vi "initErrorList.vi"(8 "error in (no error)":errorcluster, 11 "Electrometer in":refnum<class "Electrometer.lvclass">) -> (0 "error out":errorcluster, 3 "Electrometer out":refnum<class "Electrometer.lvclass">)   [LabVIEW 2016, in "Electrometer.lvclass"]
uses:
  Electrometer.lvclass
  ElectrometerConfiguration/ElectrometerInternalConfiguration.lvclass
  ElectrometerError/ElectrometerError.lvclass
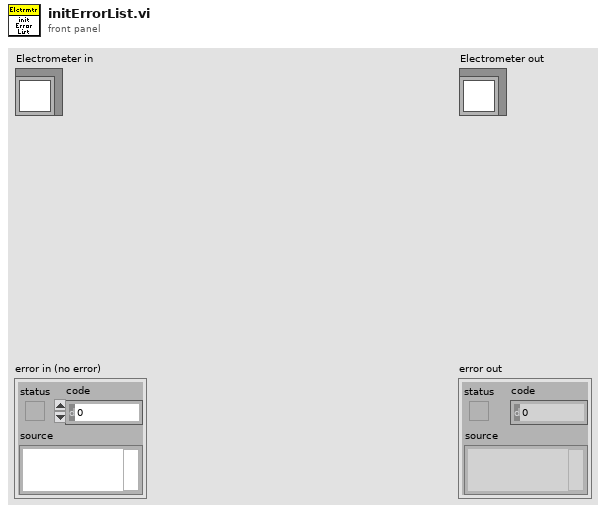
[diagram p1: front panel]
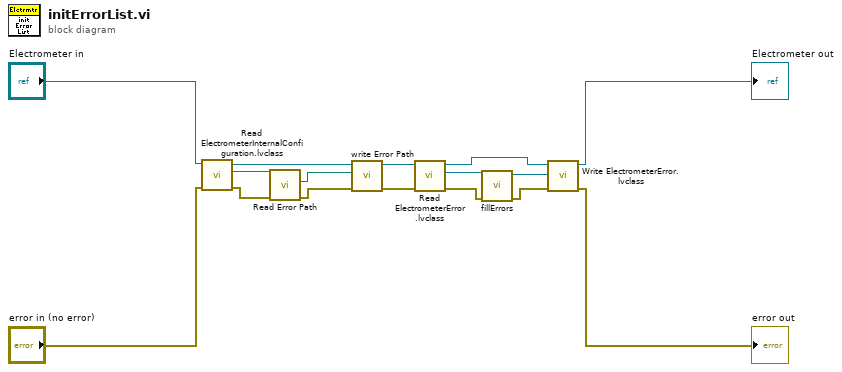
[diagram p0: block diagram]
diagram:
  n1 = call-dynamic "Read ElectrometerInternalConfiguration.lvclass.vi"("error in (no error)"="error in (no error)", "Electrometer in"="Electrometer in") -> ("error out"=w11:errorcluster, "ElectrometerInternalConfiguration.lvclass"=w15:refnum<class "ElectrometerInternalConfiguration.lvclass">, "Electrometer out"=w12:refnum<class "Electrometer.lvclass">)  [unwired: 7 in]
  n2 = call-dynamic "Read Error Path.vi"("error in (no error)"=w11, "ElectrometerInternalConfiguration in"=w15) -> ("error out"=w13:errorcluster, "Error Path"=w14:path)  [unwired: 7 in, 1 out]
  n3 = call-dynamic "write Error Path.vi"("error in (no error)"=w13, "Path"=w14, "Electrometer in"=w12) -> ("error out"=w8:errorcluster, "Electrometer out"=w9:refnum<class "Electrometer.lvclass">)  [unwired: 7 in]
  n4 = call-dynamic "Read ElectrometerError.lvclass.vi"("error in (no error)"=w8, "Electrometer in"=w9) -> ("error out"=w4:errorcluster, "ElectrometerError.lvclass"=w6:refnum<class "ElectrometerError.lvclass">, "Electrometer out"=w7:refnum<class "Electrometer.lvclass">)  [unwired: 7 in]
  n5 = call-dynamic "fillErrors.vi"("error in (no error)"=w4, "ElectrometerError in"=w6) -> ("error out"=w3:errorcluster, "ElectrometerError out"=w5:refnum<class "ElectrometerError.lvclass">)  [unwired: 8 in]
  n6 = call-dynamic "Write ElectrometerError.lvclass.vi"("error in (no error)"=w3, "ElectrometerError.lvclass"=w5, "Electrometer in"=w7) -> ("error out"=→"error out":errorcluster, "Electrometer out"=→"Electrometer out":refnum<class "Electrometer.lvclass">)  [unwired: 7 in]
